vi "INI Initialize Inifiles with Extensions.vi"(11 "Error In (no error)":errorcluster) -> (10 "Error Description File":string, 15 "Error Out":errorcluster)   [LabVIEW 2011]
doc: "This routine is used to initialize the *.ini file system, and the error management system. This is necessary for these portions of the system to function, in that it will read system file location information, and initialize globals."
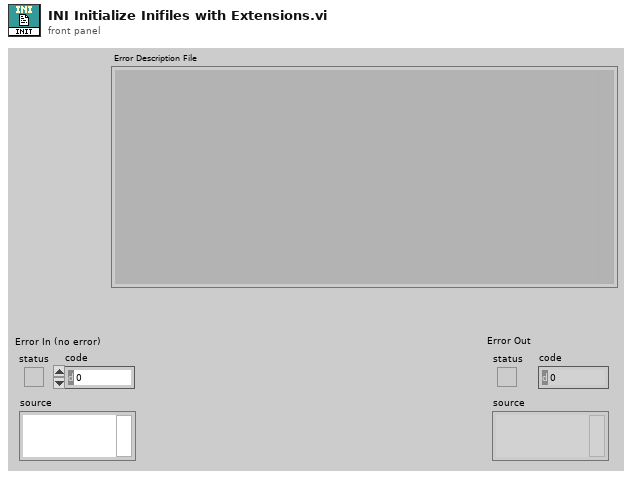
[diagram p1: front panel]
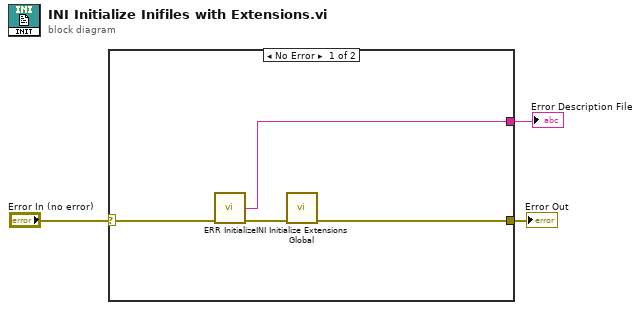
[diagram p0: block diagram]
diagram:
  n1 = case shown="No Error" "Error In (no error)" {
    selector: "Error In (no error)" -> [w4 w8]
    tunnel: [w7 w8] -> w3
    tunnel: [w5 _] -> w2
    frame No Error {
      n2 = call "ERR Initialize.vi"("Error In (no error)"=w4) -> ("Error Description File"=w5:string, "Error Out"=w6:errorcluster)  [unwired: 2 in, 11 out]
      n3 = call "INI Initialize Extensions Global.vi"("Error In (no error)"=w6) -> ("Error Out"=w7:errorcluster)  [unwired: 14 out]
    }
    frame Error {
    }
  }
  "Error Out" <- w3
  "Error Description File" <- w2
